vi "launch processes.vi"(8 "error in":errorcluster, 9 "fault list":refnum<data-value>, 10 "response fifos":T1, 11 "pool size":u8=1) -> (0 "error out":errorcluster, 3 "worker reference":T2)   [LabVIEW 2013, in "worker pool.lvlib"]
uses:
  worker pool.lvlib
  worker library reference.ctl
  worker comms.ctl
  worker commands.ctl
  request fifos.ctl
  recovery request.ctl
  <vilib>/NI/Tag Bus Module Framework/runtime/TBM module execution interface.lvclass
  <vilib>/NI/Tag Bus Module Framework/module configuration/TBM module configuration.lvclass
  rt fault.ctl
  <vilib>/NI/Tag Bus Module Framework/runtime/error classification.ctl
  response fifos.ctl
  recovery response.ctl
  <vilib>/NI/Module Execution Interface/Engine Runtime/Fault.ctl
  <vilib>/NI/Module Execution Interface/Engine Runtime/Engine Runtime Interface.lvclass
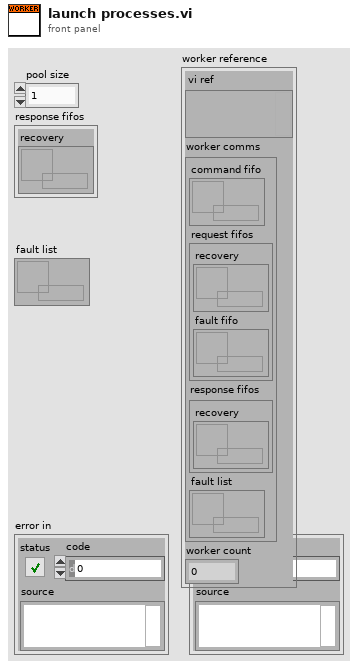
[diagram p1: front panel]
types:
  T1 = typedef "worker pool.lvlib/response fifos.ctl" = cluster{"recovery":refnum<k33>}
  T2 = typedef "worker pool.lvlib/worker library reference.ctl" = cluster{"vi ref":variant, "worker comms":T3, "worker count":i32}
  T3 = typedef "worker pool.lvlib/worker comms.ctl" = cluster{"command fifo":refnum<k33>, "request fifos":T4, "response fifos":T1, "fault list":refnum<data-value>}
  T4 = typedef "worker pool.lvlib/request fifos.ctl" = cluster{"recovery":refnum<k33>, "fault fifo":refnum<k33>}
  T5 = typedef "worker pool.lvlib/rt fault.ctl" = cluster{"code":i32, "classification":T6, "iteration":u64, "cfg ref":refnum<data-value>}
  T6 = typedef "TBM module execution interface.lvclass/error classification.ctl" = enum16{"unknown", "none", "trivial", "recoverable", "critical"}
  T7 = typedef "worker pool.lvlib/worker commands.ctl" = enum16{"shutdown", "recover module", "record fault"}
  T8 = typedef "worker pool.lvlib/recovery request.ctl" = cluster{"module ref":refnum<data-value>, "engine reference":i32, "original run flags":u8, "attempts allowed":u16, "cfg ref":refnum<data-value>}
  T9 = cluster{"read mode":enum16{"polling", "blocking"}, "write mode":enum16{"polling", "blocking"}}
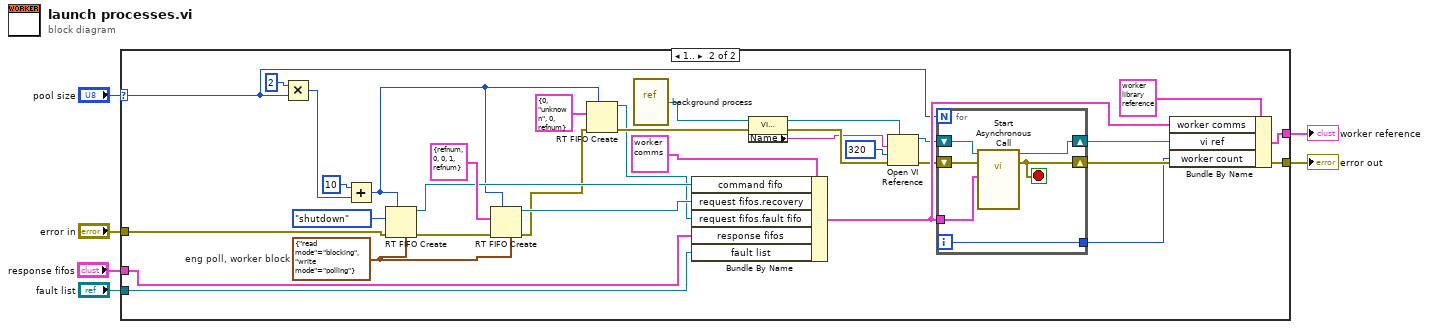
[diagram p0: block diagram]
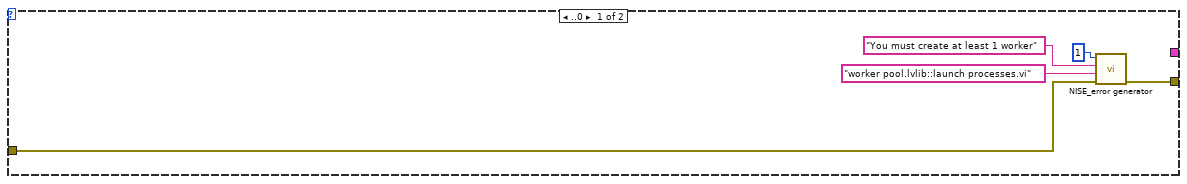
[diagram p2: hidden frame]
diagram:
  n1 = case shown="1.." "pool size" {
    selector: "pool size" -> [_ w29]
    tunnel: "error in" -> [w11 w42]
    tunnel: [w10 w40] -> w5
    tunnel: [_ w38] -> w3
    tunnel: "response fifos" -> [_ w35]
    tunnel: "fault list" -> [_ w25]
    frame ..0 {
      n2 = call <vilib>:"NISE_error generator.vi"("error in"=w11, "source"="worker pool.lvlib::launch processes.vi", "append error message"="You must create at least 1 worker", "error code (0)"=1) -> ("error out"=w10:errorcluster)  [unwired: 5 in]
    }
    frame 1.. {
      w30 = T9 {"read mode"=enum."blocking", "write mode"=enum."polling"}  # eng poll, worker block
      n3 = Multiply(x=u8 2, y=w29) -> (x*y=w27:u8)
      n4 = Add(x=u8 10, y=w27) -> (x+y=w23:u8)
      n5 = RT FIFO Create(1:worker_commands."shutdown" ("worker actions"), 3:w42, 4:w23, 7:w30) -> (8:w32:refnum<k33>, 11:w36:errorcluster)  [unwired: 4 in, 1 out]
      n6 = RT FIFO Create(1:T8 {"module ref"=refnum, "engine reference"=0, "original run flags"=0, "attempts allowed"=1, "cfg ref"=refnum} ("recovery request"), 3:w36, 4:w23, 7:w30) -> (8:w34:refnum<k33>, 11:w24:errorcluster)  [unwired: 4 in, 1 out]
      n7 = RT FIFO Create(1:T5 {"code"=0, "classification"=enum."unknown", "iteration"=0, "cfg ref"=refnum} ("rt fault"), 3:w24, 4:w23) -> (8:w21:refnum<k33>, 11:w22:errorcluster)  [unwired: 5 in, 1 out]
      n8 = vi-ref "background process.vi"() -> (w43:refnum<vi>)
      n9 = Bundle By Name(cluster=T3 {"command fifo"=refnum, "request fifos"={"recovery"=refnum, "fault fifo"=refnum}, "response fifos"={"recovery"=refnum}, "fault list"=refnum} ("worker comms"), "command fifo"=w32, "request fifos.recovery"=w34, "request fifos.fault fifo"=w21, "response fifos"=w35, "fault list"=w25) -> (w37:T3)
      n10 = property class="VI (strict)"(reference=w43, error in=w22) -> (reference out=w16:refnum<vi>, error out=w18:errorcluster, "Name"=w17:string)
      n11 = Open VI Reference(type specifier VI Refnum (for type only)=w16, vi path=w17, options=320, error in (no error)=w18) -> (vi reference=w14:refnum<vi>, error out=w19:errorcluster)  [unwired: 2 in]
      n12 = for {
        N: w29 -> [_]
        tunnel: w37 -> [w45]
        shift-right: [w46] -> w40
        shift-left: w19 -> [w49]
        shift-right: [w47] -> w13
        shift-left: w14 -> [w48]
        tunnel: [w44] -> w12
        i -> [w44]
        stop <- w46 stop-if-true
        n13 = call-by-ref "Start Asynchronous Call"(reference=w48, error in=w49, "communication refs"=w45) -> (reference out=w47:refnum<vi>, error out=w46:errorcluster)  [unwired: 11 in]
      }
      n14 = Bundle By Name(cluster=T2 {"vi ref"=variant, "worker comms"={"command fifo"=refnum, "request fifos"={"recovery"=refnum, "fault fifo"=refnum}, "response fifos"={"recovery"=refnum}, "fault list"=refnum}, "worker count"=0} ("worker library"), "worker comms"=w37, "vi ref"=w13, "worker count"=w12) -> (w38:T2)
    }
  }
  "error out" <- w5
  "worker reference" <- w3
